vi "CRYPEAQ DFTFrame.vi"(8 "NF":dbl=2048.0, 10 "Fs":dbl=44100.0, 11 "x":dbl[](array[numeric])) -> (0 "Freq(Hz)":dbl[](array[numeric]), 2 "hw":dbl[](array[numeric]), 3 "X2":dbl[](array[numeric]))   [LabVIEW 2013]
panel:
  out "Waveform Graph":dbl[](graph)
  out "XY Graph":cluster{dbl[], "X2":dbl[]}(graph)
  in  "Amax":dbl=32768.0
  in  "Lp":dbl=92.0
  in  "fc":dbl=1019.5
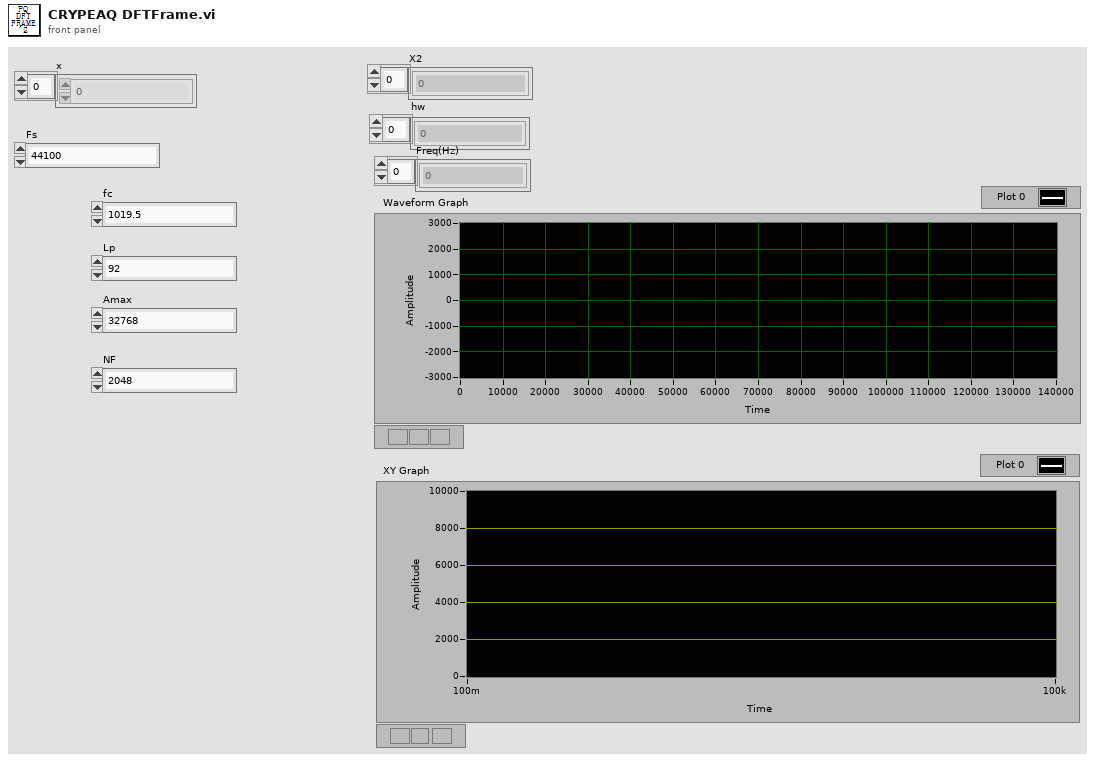
[diagram p1: front panel]
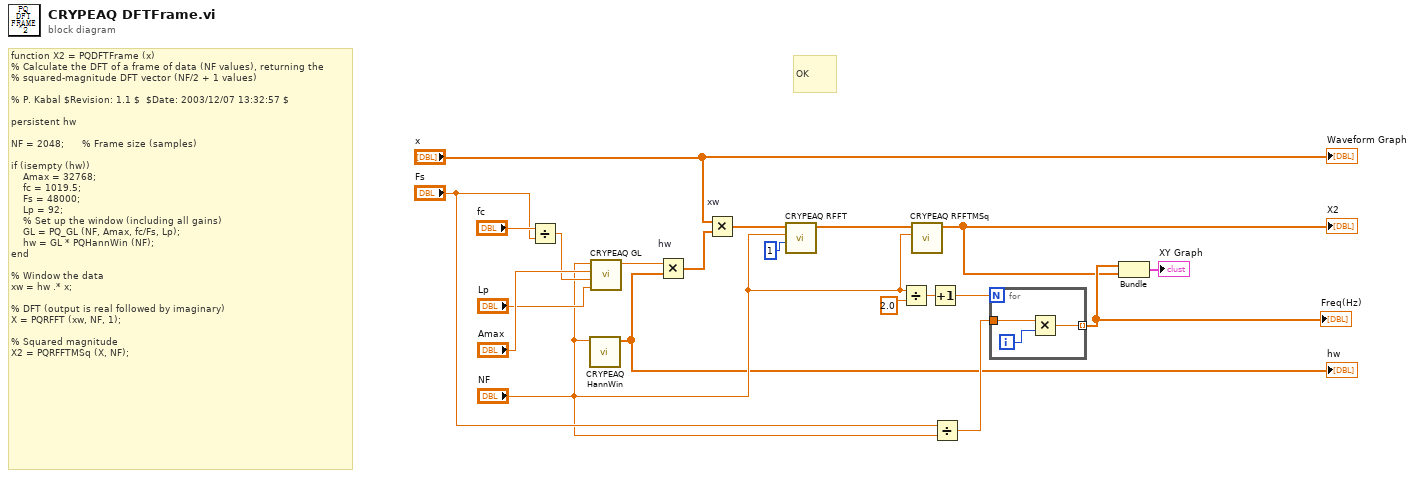
[diagram p0: block diagram]
diagram:
  # "OK"
  # "function X2 = PQDFTFrame (x)\n% Calculate the DFT of a frame of data (NF values), returning the\n% squared-magnitude DFT vector (NF/2 + 1 values)\n\n% P. Kabal $Revision: 1.1 $  $Date: 2003/12/07 13:32:57 $\n\npersistent hw\n\nNF = 2048;      % Frame size (samples)\n\nif (isempty (hw))\n    Amax = 32768;\n    fc = 1019.5;\n    Fs = 48000;\n    Lp = 92;\n    % Set up the window (including all gains)\n    GL = PQ_GL (NF, Amax, fc/Fs, Lp);\n    hw = GL * PQHannWin (NF);\nend\n\n% Window the data\nxw = hw .* x;\n\n% DFT (output is real followed by imaginary)\nX = PQRFFT (xw, NF, 1);\n\n% Squared magnitude\nX2 = PQRFFTMSq (X, NF);"
  n1 = Divide(x="fc", y="Fs") -> (x/y=w18:dbl)
  n2 = call "CRYPEAQ HannWin.vi"("NF"="NF") -> ("hw"=w4:dbl[])  [unwired: 10 in]
  "hw" <- w4
  n3 = call "CRYPEAQ GL.vi"("Lp"="Lp", "fcN"=w18, "Amax"="Amax", "NF"="NF") -> ("GL"=w16:dbl)  [unwired: 7 in]
  n4 = Multiply "hw"(x=w16, y=w4) -> (x*y=w15:dbl[])
  n5 = Multiply "xw"(x="x", y=w15) -> (x*y=w3:dbl[])
  n6 = call "CRYPEAQ RFFT.vi"("ifn"=1, "N"="NF", "x"=w3) -> ("X"=w2:dbl[])  [unwired: 8 in]
  n7 = Divide(x="NF", y=2.0) -> (x/y=w13:dbl)
  n8 = call "CRYPEAQ RFFTMSq.vi"("N"="NF", "X"=w2) -> ("X2"=w1:dbl[])  [unwired: 9 in]
  "X2" <- w1
  n9 = Increment(x=w13) -> (x+1=w8:dbl)
  n10 = Divide(x="Fs", y="NF") -> (x/y=w11:dbl)
  n11 = for {
    N: w8 -> [_]
    tunnel: w11 -> [w22]
    tunnel: [w21] -> w10 mode=indexing
    i -> [w23]
    n12 = Multiply(x=w22, y=w23) -> (x*y=w21:dbl)
  }
  "Freq(Hz)" <- w10
  n13 = Bundle(w10, "X2"=w1) -> (→"XY Graph":cluster{dbl[], "X2":dbl[]})  [unwired: 1 in]
  "Waveform Graph" <- "x"
